vi "Get IConfiguration.vi"(8 "error in":errorcluster, 11 "IHasConfiguration in":refnum<class "IHasConfiguration.lvclass">) -> (0 "error out":errorcluster, 2 "IConfiguration":refnum<class "IConfiguration.lvclass">, 3 "IHasConfiguration out":refnum<class "IHasConfiguration.lvclass">)   [LabVIEW 2024, in "IHasConfiguration.lvclass"]
uses:
  IHasConfiguration.lvclass
  IConfiguration/IConfiguration.lvclass
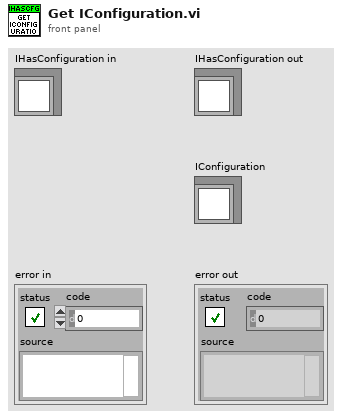
[diagram p1: front panel]
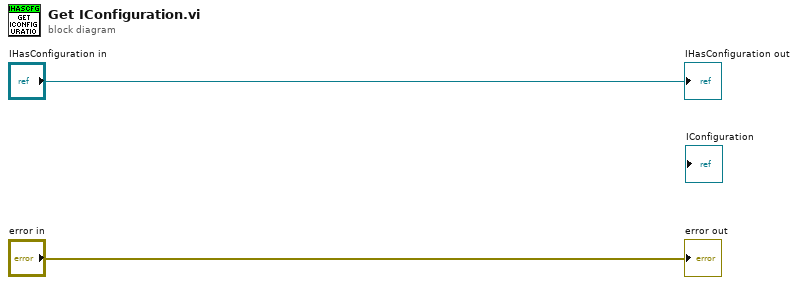
[diagram p0: block diagram]
diagram:
  "error out" <- "error in"
  "IHasConfiguration out" <- "IHasConfiguration in"
